vi "GlobalDataNames7.vi"(2 "Data  Names In":string[](array[string]), 3 "Data Name In":string, 4 "Element #":u16, 5 "Function select":string) -> (0 "Data Names Out":string[](array[string]), 1 "Data Name Out":string)   [LabVIEW 2013]
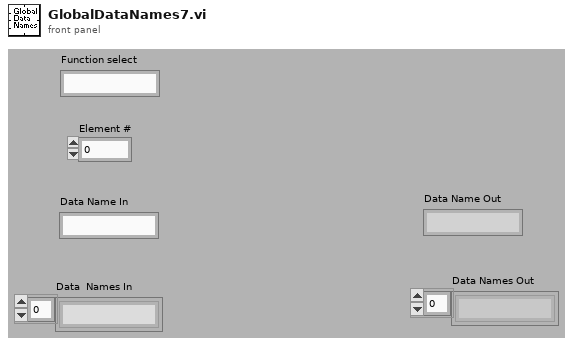
[diagram p1: front panel]
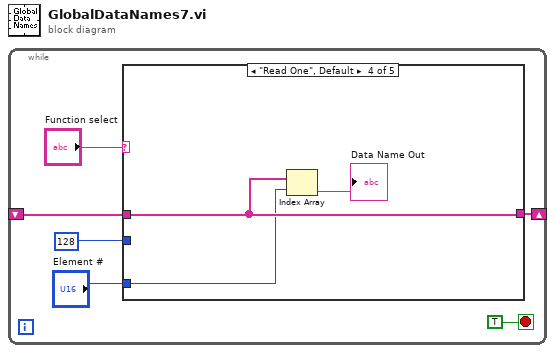
[diagram p0: block diagram]
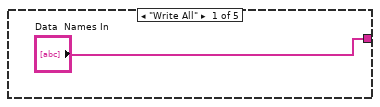
[diagram p2: hidden frame]
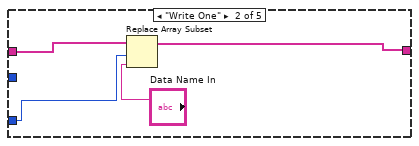
[diagram p3: hidden frame]
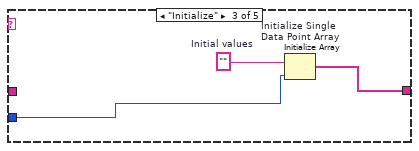
[diagram p4: hidden frame]
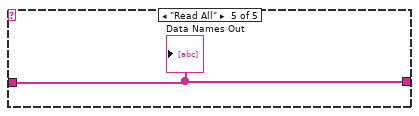
[diagram p5: hidden frame]
diagram:
  n1 = while {
    shift-right: [w4] -> _
    shift-left: _ -> [w3]
    stop <- TRUE stop-if-true
    n2 = case shown="\"Read One\", Default" "Function select" {
      tunnel: 128 -> [_ _ w14 _ _]
      tunnel: ["Data  Names In" w10 w12 w16 w18] -> w4
      tunnel: w3 -> [_ w11 _ w16 w18]
      tunnel: "Element #" -> [_ w8 _ w15 _]
      frame "Write All" {
      }
      frame "Write One" {
        n3 = Replace Array Subset(array=w11, new element="Data Name In", index=w8) -> (w10:string[])
      }
      frame "Initialize" {
        w13 = ""  # Initial values
        n4 = Initialize Array "Initialize Single\nData Point Array"(w13, w14) -> (w12:string[])
      }
      frame "Read One", Default {
        n5 = Index Array(array=w16, index=w15) -> (element=→"Data Name Out":string)
      }
      frame "Read All" {
        "Data Names Out" <- w18
      }
    }
  }
